vi "Tochka.vi"() -> ()   [LabVIEW 2011]
uses:
  ChT.ctl
panel:
  in  "T":refnum<user-event>
  out "32bit integer":i32
  in  "stop":bool
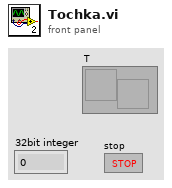
[diagram p1: front panel]
types:
  T1 = typedef "ChT.ctl" = enum16{"Random", "Stop"}
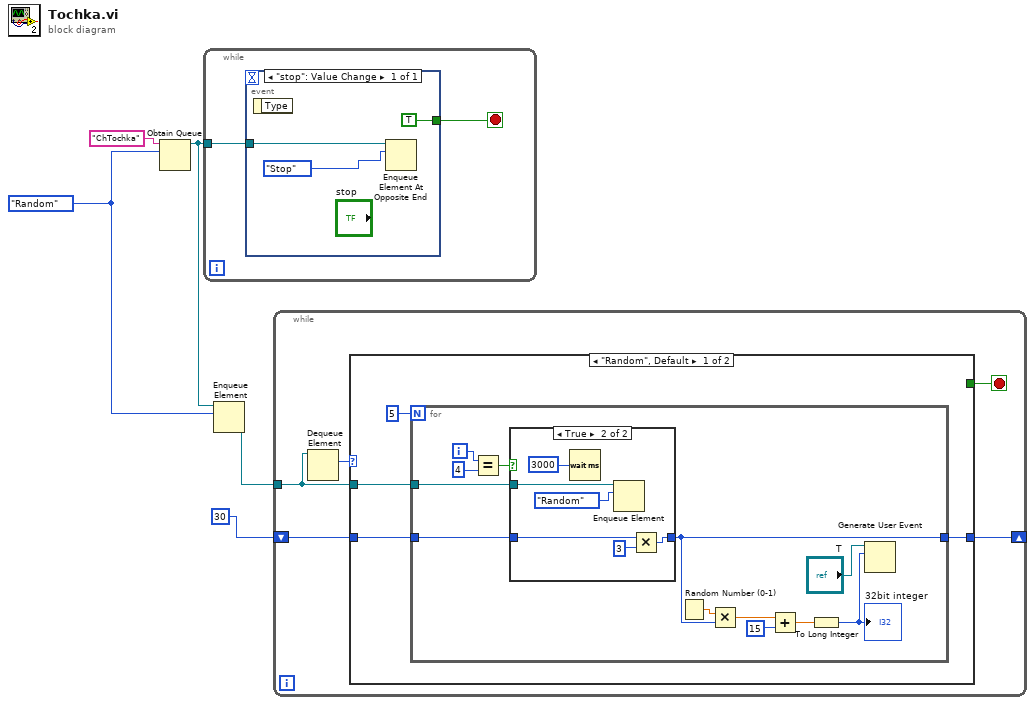
[diagram p0: block diagram]
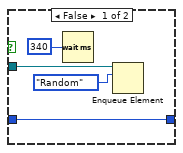
[diagram p2: hidden frame]
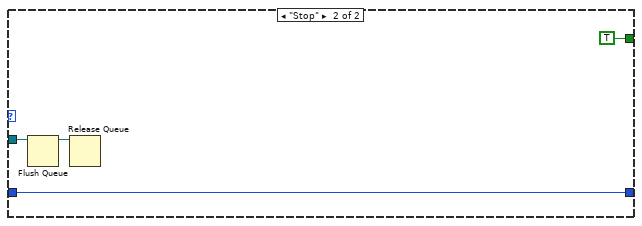
[diagram p3: hidden frame]
diagram:
  w2 = ChT."Random" ("Enum")
  n1 = Obtain Queue(name (unnamed)="ChTochka", element data type=w2) -> (queue out=w5:refnum<queue>)  [unwired: 3 in, 2 out]
  n2 = while {
    tunnel: w5 -> [w7]
    stop <- w6 stop-if-true
    n3 = event shown="[0] \"stop\": Value Change" {
      selector: _ -> [_]
      dyn-events: _ -> [_]
      timeout: _ -> [_]
      tunnel: w7 -> [w10]
      tunnel: [TRUE] -> w6
      event "stop": Value Change {
        n4 = event-data() -> ()  [unwired: 1 in, 1 out]
        n5 = Enqueue Element At Opposite End(queue=w10, element=ChT."Stop" ("Enum")) -> ()  [unwired: 2 in, 3 out]
      }
    }
  }
  n6 = Enqueue Element(queue=w5, element=w2) -> (queue out=w3:refnum<queue>)  [unwired: 2 in, 2 out]
  n7 = while {
    tunnel: w3 -> [w14]
    shift-right: [w11] -> _
    shift-left: u32 30 ("y") -> [w12]
    stop <- w13 stop-if-true
    n8 = Dequeue Element(queue=w14) -> (element=w15:T1)  [unwired: 2 in, 3 out]
    n9 = case shown="\"Random\", Default" w15 {
      tunnel: [_ TRUE] -> w13
      tunnel: w14 -> [w19 w43]
      tunnel: w12 -> [w17 w42]
      tunnel: [w16 w42] -> w11
      frame "Random", Default {
        n10 = for {
          N: 5 -> [_]
          tunnel: w19 -> [w28]
          tunnel: w17 -> [w21]
          tunnel: [w20] -> w16
          i -> [w30]
          n11 = Equal?(x=w30, y=4) -> (x = y?=w29:bool)
          n12 = case shown="True" w29 {
            tunnel: w28 -> [w34 w39]
            tunnel: w21 -> [w32 w38]
            tunnel: [w32 w37] -> w20
            frame False {
              n13 = Wait (ms)(milliseconds to wait=u32 340) -> ()  [unwired: 1 out]
              n14 = Enqueue Element(queue=w34, element=enum16{"Random", "Stop"}."Random" ("Enum")) -> ()  [unwired: 2 in, 3 out]
            }
            frame True {
              n15 = Wait (ms)(milliseconds to wait=u32 3000) -> ()  [unwired: 1 out]
              n16 = Enqueue Element(queue=w39, element=enum16{"Random", "Stop"}."Random" ("Enum")) -> ()  [unwired: 2 in, 3 out]
              n17 = Multiply(x=w38, y=u32 3) -> (x*y=w37:u32)
            }
          }
          n18 = Random Number (0-1)() -> (number: 0 to 1=w24:dbl)
          n19 = Multiply(x=w24, y=w20) -> (x*y=w25:dbl)
          n20 = Add(x=w25, y=15) -> (x+y=w27:dbl)
          n21 = To Long Integer(number=w27) -> (32bit integer=w23:i32)
          "32bit integer" <- w23
          n22 = Generate User Event(user event="T", event data cluster=w23) -> ()  [unwired: 1 in, 2 out]
        }
      }
      frame "Stop" {
        n23 = Flush Queue(queue=w43) -> (queue out=w44:refnum<queue>)  [unwired: 1 in, 2 out]
        n24 = Release Queue(queue=w44) -> ()  [unwired: 2 in, 3 out]
      }
    }
  }
